vi "Edit Substeps Analog Input.vi"(0 "Sequence Context In":refnum<k7>, 5 "AIRead":T1, 11 "error in":errorcluster) -> (4 "Report Text":string, 6 "AIReadOut":T1, 15 "error out":errorcluster)   [LabVIEW 2023, in "LTT_TeststandSteptypes.lvlib"]
doc: "This VI Analog Input Signal Map and Multinumberic Edit Sub step"
uses:
  LTT_TeststandSteptypes.lvlib
  HardwareAbstractionLayer_LVOOP/Database/SQL Public VI/Control/DB Options.ctl
  <vilib>/addons/TestStand/_TSUtility.llb/TestStand - Start Modal Dialog (Sequence Context).vi
  <vilib>/addons/TestStand/_TSUtility.llb/TestStand - End Modal Dialog (Sequence Context).vi
  HardwareAbstractionLayer_LVOOP/Database/Database.lvclass
panel:
  in  "Close":bool
  in  "OK":bool
  in  "Station No":i32
  in  "Signal Name":string(combo)
  in  "Signal Name List":string[](array[combo])
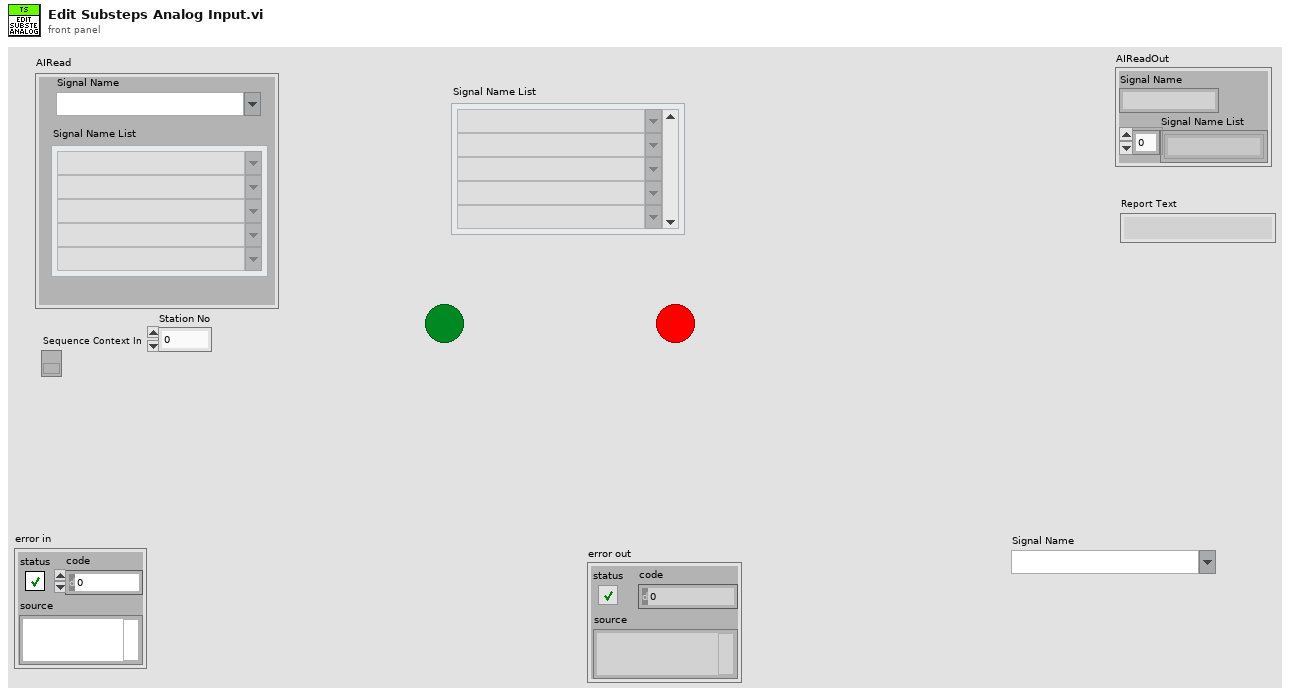
[diagram p1: front panel]
types:
  T1 = cluster{"Signal Name":string, "Signal Name List":string[]}
  T2 = typedef "HardwareAbstractionLayer_LVOOP.lvlib/Database.lvclass/DB Options.ctl" = enum16{"Init", "Select Data", "Insert Data", "Update Data", "Delete Data", "Execute Query", "Create Schema", "Create Table", "List Tables", "List Columns", "Close"}
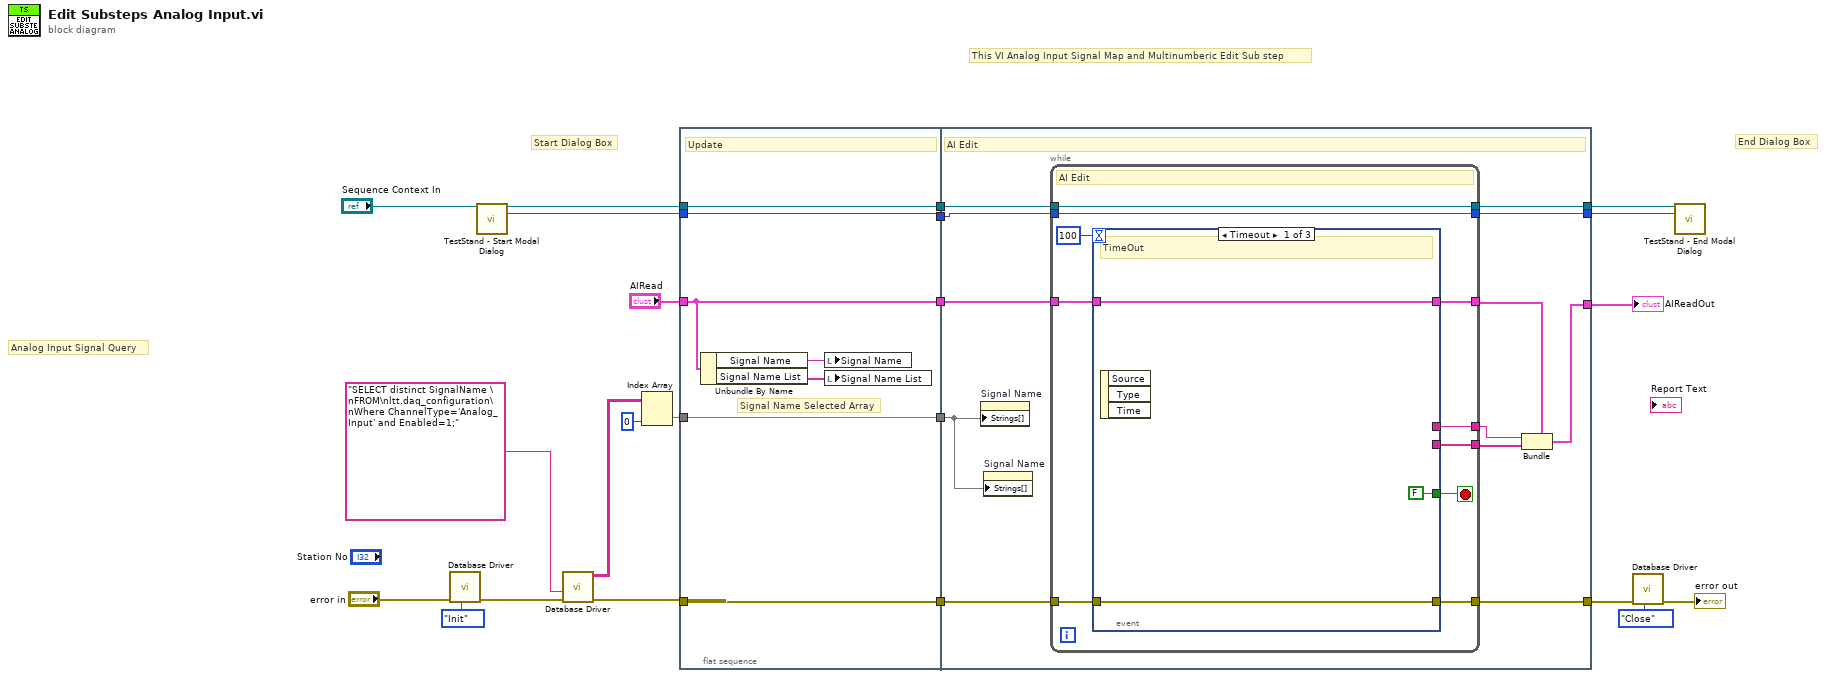
[diagram p0: block diagram]
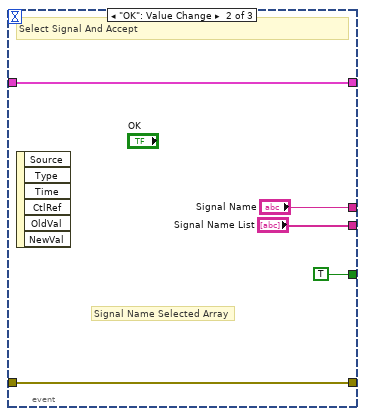
[diagram p2: hidden frame]
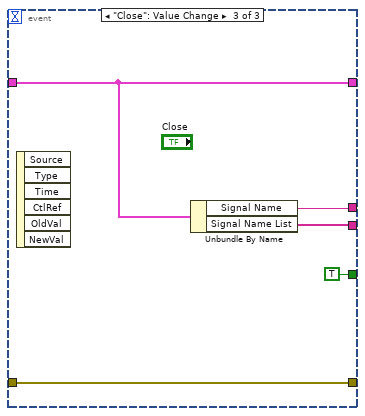
[diagram p3: hidden frame]
diagram:
  # "Analog Input Signal Query"
  # "This VI Analog Input Signal Map and Multinumberic Edit Sub step"
  # "End Dialog Box"
  # "Start Dialog Box"
  n1 = call "Database Driver.vi"("Options"=DB_Options."Init", "error in"="error in") -> ("error out"=w5:errorcluster)  [unwired: 6 in, 3 out]
  n2 = call-poly <vilib>:"TestStand - Start Modal Dialog.vi"("Sequence Context In"="Sequence Context In") -> ("Sequence Context Out"=w16:refnum<k7>, "Modal ID"=w15:i32)  [unwired: 10 in, 3 out]
  n3 = call "Database Driver.vi"("error in"=w5, "SQL query"="SELECT distinct SignalName \nFROM\nltt.daq_configuration\nWhere ChannelType='Analog_Input' and Enabled=1;") -> ("error out"=w7:errorcluster, "data"=w10:string[][])  [unwired: 6 in, 2 out]
  n4 = Index Array(array=w10, index (col)=0 ("disabled index (col)")) -> (element=w8:string[])  [unwired: 1 in]
  n5 = flat-sequence {
    tunnel: "AIRead" -> [w30]
    tunnel: [w30] -> w23
    tunnel: w7 -> [w27]
    tunnel: [w27] -> w20
    tunnel: w8 -> [w26]
    tunnel: [w26] -> w18
    tunnel: w16 -> [w25]
    tunnel: w15 -> [w24]
    tunnel: [w25] -> w14
    tunnel: [w24] -> w13
    tunnel: w23 -> [w37]
    tunnel: [w42] -> w21
    tunnel: w20 -> [w39]
    tunnel: [w38] -> w19
    tunnel: w18 -> [w35]
    tunnel: w14 -> [w34]
    tunnel: [w33] -> w12
    tunnel: w13 -> [w32]
    tunnel: [w31] -> w11
    frame #0 {
      # "Signal Name Selected Array"
      # "Update"
      n6 = Unbundle By Name(w30) -> ("Signal Name"=w29:string, "Signal Name List"=w28:string[])
      n7 = local write "Signal Name"(w29) -> ()
      n8 = local write "Signal Name List"(w28) -> ()
    }
    frame #1 {
      # "AI Edit"
      n9 = property on="Signal Name" class="CmbBox"("Strings[]"=w35) -> ()  [unwired: 2 in, 2 out]
      n10 = property on="Signal Name" class="CmbBox"("Strings[]"=w35) -> ()  [unwired: 2 in, 2 out]
      n11 = while {
        tunnel: [w52] -> w41
        tunnel: [w51] -> w40
        tunnel: w39 -> [w47]
        tunnel: [w46] -> w38
        tunnel: w37 -> [w45]
        tunnel: [w44] -> w36
        tunnel: w34 -> [w50]
        tunnel: [w50] -> w33
        tunnel: w32 -> [w49]
        tunnel: [w49] -> w31
        stop <- w43 stop-if-true
        # "AI Edit"
        n12 = event shown="[0] Timeout" {
          selector: _ -> [_ _ _]
          dyn-events: _ -> [_ _ _]
          timeout: 100 -> [_ _ _]
          tunnel: [_ "Signal Name" w64] -> w52
          tunnel: [_ "Signal Name List" w63] -> w51
          tunnel: w47 -> [w54 w58 w61]
          tunnel: [w54 w58 w61] -> w46
          tunnel: w45 -> [w55 w57 w65]
          tunnel: [w55 w57 w65] -> w44
          tunnel: [FALSE TRUE TRUE] -> w43
          event Timeout {
            # "TimeOut"
            n13 = event-data() -> ()  [unwired: 1 in, 3 out]
          }
          event "OK": Value Change {
            # "Signal Name Selected Array"
            # "Select Signal And Accept"
            n14 = event-data() -> ()  [unwired: 1 in, 6 out]
          }
          event "Close": Value Change {
            n15 = event-data() -> ()  [unwired: 1 in, 6 out]
            n16 = Unbundle By Name(w65) -> ("Signal Name"=w64:string, "Signal Name List"=w63:string[])
          }
        }
      }
      n17 = Bundle(cluster=w36, "Signal Name"=w41, "Signal Name List"=w40) -> (w42:T1)
    }
  }
  n18 = call "Database Driver.vi"("Options"=DB_Options."Close", "error in"=w19) -> ("error out"=→"error out":errorcluster)  [unwired: 6 in, 3 out]
  n19 = call-poly <vilib>:"TestStand - End Modal Dialog.vi"("Sequence Context In"=w12, "Modal ID"=w11) -> ()  [unwired: 13 in, 1 out]
  "AIReadOut" <- w21
